vi "Barycen.vi"(7 "Array":i32[][](array[numeric])) -> (6 "X?":dbl, 10 "Y?":dbl)   [LabVIEW 2019]
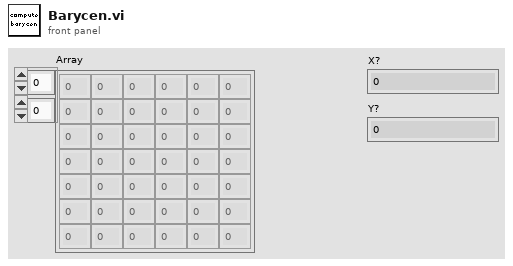
[diagram p1: front panel]
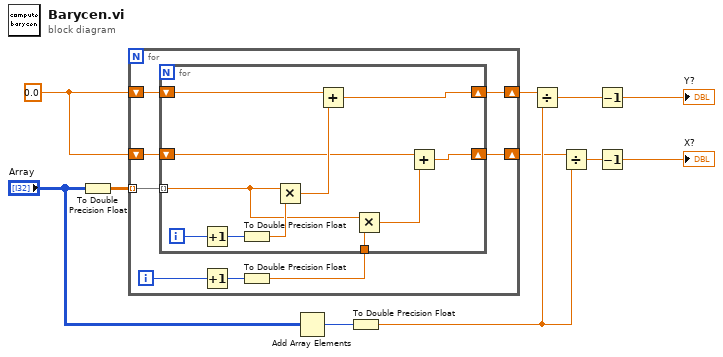
[diagram p0: block diagram]
diagram:
  w8 = 0.0
  n1 = To Double Precision Float(number="Array") -> (double precision float=w11:dbl[][])
  n2 = for {
    tunnel: w11 -> [w19] mode=indexing
    shift-right: [w13] -> w7
    shift-left: w8 -> [w18]
    shift-right: [w12] -> w6
    shift-left: w8 -> [w17]
    i -> [w15]
    n3 = Increment(x=w15) -> (x+1=w14:i32)
    n4 = To Double Precision Float(number=w14) -> (double precision float=w16:dbl)
    n5 = for {
      tunnel: w19 -> [w20] mode=indexing
      tunnel: w16 -> [w29]
      shift-right: [w23] -> w13
      shift-left: w18 -> [w26]
      shift-right: [w22] -> w12
      shift-left: w17 -> [w24]
      i -> [w28]
      n6 = Increment(x=w28) -> (x+1=w27:i32)
      n7 = To Double Precision Float(number=w27) -> (double precision float=w30:dbl)
      n8 = Multiply(x=w20, y=w30) -> (x*y=w25:dbl)
      n9 = Add(x=w26, y=w25) -> (x+y=w23:dbl)
      n10 = Multiply(x=w20, y=w29) -> (x*y=w21:dbl)
      n11 = Add(x=w24, y=w21) -> (x+y=w22:dbl)
    }
  }
  n12 = Add Array Elements(numeric array="Array") -> (sum=w10:i32)
  n13 = To Double Precision Float(number=w10) -> (double precision float=w9:dbl)
  n14 = Divide(x=w7, y=w9) -> (x/y=w5:dbl)
  n15 = Divide(x=w6, y=w9) -> (x/y=w4:dbl)
  n16 = Decrement(x=w5) -> (x-1=→"Y?":dbl)
  n17 = Decrement(x=w4) -> (x-1=→"X?":dbl)
